vi "Configure Math.vi"   [LabVIEW 2011, in "Tektronix 7000 Series.lvlib"]
doc: "This polymorphic VI configures math channel with different math operations.\n\nThe Configure Math (Basic) VI configures a math channel for standard waveform math operations such as add, subtract, multiply, and divide.\n\nThe Configure Math (Advanced) VI configures a math channel using a mathematical expression."
uses:
  Tektronix 7000 Series.lvlib
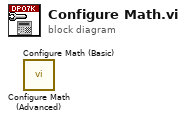
[diagram p0: block diagram]
diagram:
  n1 = call "Configure Math (Advanced).vi"() -> ()  [unwired: 10 in, 2 out]
  n2 = call "Configure Math (Basic).vi"() -> ()  [unwired: 10 in, 2 out]
